vi "Timestamp to Unix ns.vi"(3 "Time Stamp":timestamp) -> (1 "unix ns":i64)   [LabVIEW 2020, in "Vecto.lvlib"]
uses:
  Vecto.lvlib
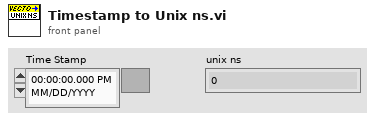
[diagram p1: front panel]
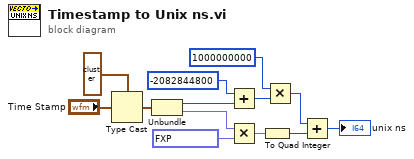
[diagram p0: block diagram]
diagram:
  n1 = Type Cast(type=cluster{i64, "Numeric":fxp<+,64,0>} {0, "Numeric"=0.0}, x="Time Stamp") -> (*(type *) &x=w12:cluster{i64, "Numeric":fxp<+,64,0>})
  n2 = Unbundle(w12) -> (w4:i64, "Numeric"=w5:fxp<+,64,0>)
  n3 = Add(x=i64 -2082844800 ("y"), y=w4) -> (x+y=w2:i64)
  n4 = Multiply(x=w5, y=fxp<+,21,30> 1000000000.0) -> (x*y=w10:fxp<+,64,30>)
  n5 = To Quad Integer(1:w10) -> (0:w9:i64)
  n6 = Multiply(x=i64 1000000000, y=w2) -> (x*y=w8:i64)
  n7 = Add(x=w8, y=w9) -> (x+y=→"unix ns":i64)
